vi "CalulateSpeed.vi"(8 "D":dbl, 9 "C":dbl, 10 "B":dbl, 11 "A":dbl) -> (0 "wheelSpeed4":dbl, 1 "wheelSpeed3":dbl, 2 "wheelSpeed2":dbl, 3 "wheelSpeed1":dbl)   [LabVIEW 2019]
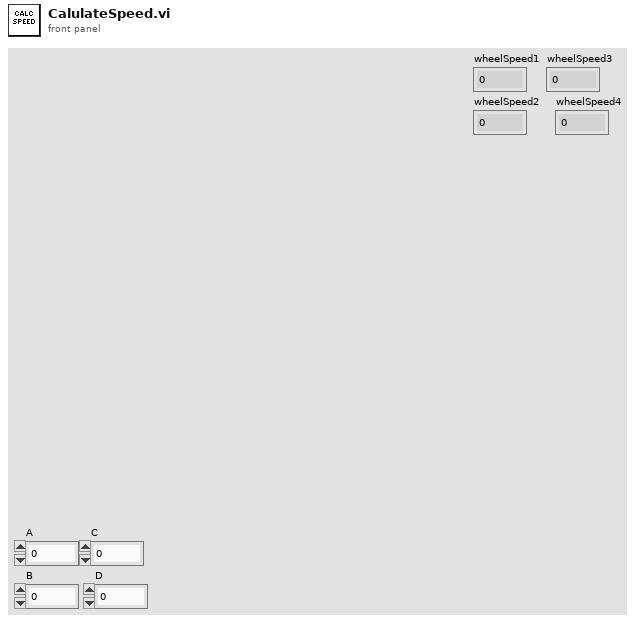
[diagram p1: front panel]
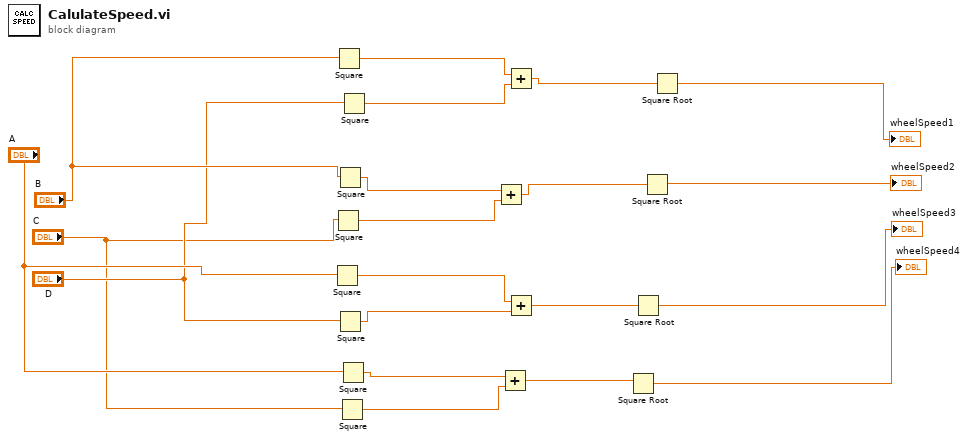
[diagram p0: block diagram]
diagram:
  n1 = Square(x="A") -> (x^2=w13:dbl)
  n2 = Square(x="C") -> (x^2=w15:dbl)
  n3 = Square(x="B") -> (x^2=w20:dbl)
  n4 = Square(x="B") -> (x^2=w16:dbl)
  n5 = Square(x="D") -> (x^2=w12:dbl)
  n6 = Square(x="C") -> (x^2=w8:dbl)
  n7 = Square(x="A") -> (x^2=w9:dbl)
  n8 = Square(x="D") -> (x^2=w19:dbl)
  n9 = Add(x=w16, y=w15) -> (x+y=w14:dbl)
  n10 = Add(x=w9, y=w8) -> (x+y=w7:dbl)
  n11 = Add(x=w20, y=w19) -> (x+y=w18:dbl)
  n12 = Add(x=w13, y=w12) -> (x+y=w11:dbl)
  n13 = Square Root(x=w7) -> (sqrt(x)=→"wheelSpeed4":dbl)
  n14 = Square Root(x=w11) -> (sqrt(x)=→"wheelSpeed3":dbl)
  n15 = Square Root(x=w14) -> (sqrt(x)=→"wheelSpeed2":dbl)
  n16 = Square Root(x=w18) -> (sqrt(x)=→"wheelSpeed1":dbl)
